vi "Read Last Average.vi"(11 "Timed Average Buffer":T1) -> (0 "error IO":errorcluster, 2 "Last Average":dbl)   [LabVIEW 2015, in "TimedAverageBuffer.lvlib" / "TimedAverageBuffer.lvclass"]
uses:
  TimedAverageBuffer.lvclass
  TimedAverageBuffer Reference.ctl
  TimedAverageBuffer.lvclass/TimedAverageBuffer.ctl
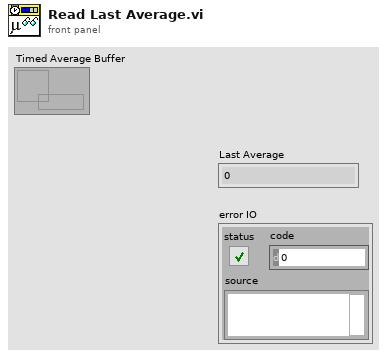
[diagram p1: front panel]
types:
  T1 = typedef "TimedAverageBuffer.lvlib/TimedAverageBuffer.lvclass/TimedAverageBuffer Reference.ctl" = refnum<data-value>
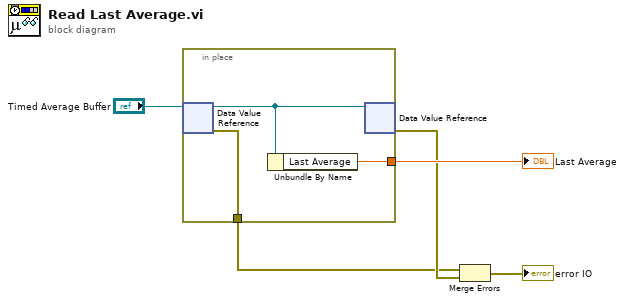
[diagram p0: block diagram]
diagram:
  n1 = in-place {
    in-place-border: [w8] -> w4
    in-place-border: [w6] -> w1
    n2 = in-place-dvr #1("Timed Average Buffer") -> (w7:refnum<class "TimedAverageBuffer.lvclass">, w6:errorcluster)
    n3 = Unbundle By Name(w7) -> ("Last Average"=w8:dbl)
    n4 = in-place-dvr #1(w7) -> (w3:errorcluster)  [unwired: 1 out]
  }
  "Last Average" <- w4
  n5 = Merge Errors(w1, w3) -> (→"error IO":errorcluster)
